vi "Toggle Channel.vi"(8 "error in":errorcluster, 9 "State":bool, 10 "Name":string, 11 "MLTFNC in":refnum<class "MLTFNC.lvclass">) -> (0 "error out":errorcluster, 3 "MLTFNC out":refnum<class "MLTFNC.lvclass">)   [LabVIEW 2019, in "MLTFNC.lvlib" / "MLTFNC.lvclass"]
doc: "This parent method must be called first,\nIt searches for the literal string name of the channel and stores the array index of the literal string if present, or returns an error if the channel is not found."
uses:
  Library/MLTFNC.lvclass
  C:/Users/Public/Documents/Development/builds/Instruments/Instruments.lvlibp/Library/Instruments.lvclass
  builds/Instruments/Instruments.lvlibp/Private/Polymorphic/Special/Event from String.vi
  builds/Instruments/Instruments.lvlibp/Accessors/Command with Logging.vi
  builds/Instruments/Instruments.lvlibp/Library/Instruments.lvclass
  builds/Instruments/Instruments.lvlibp
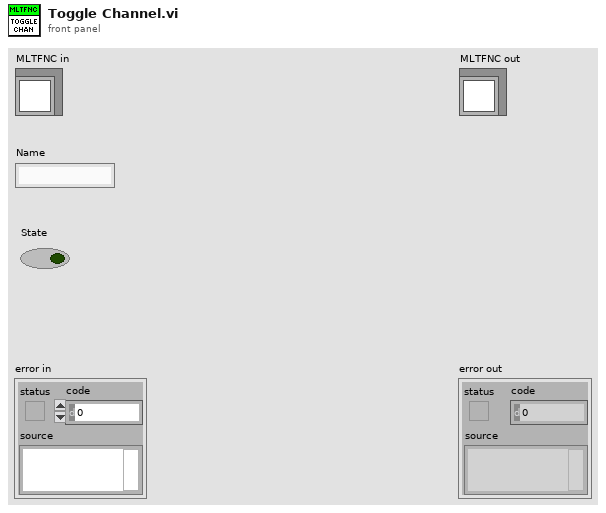
[diagram p1: front panel]
types:
  T1 = cluster{"Timestamp":timestamp, "Description":string, "Data":string}
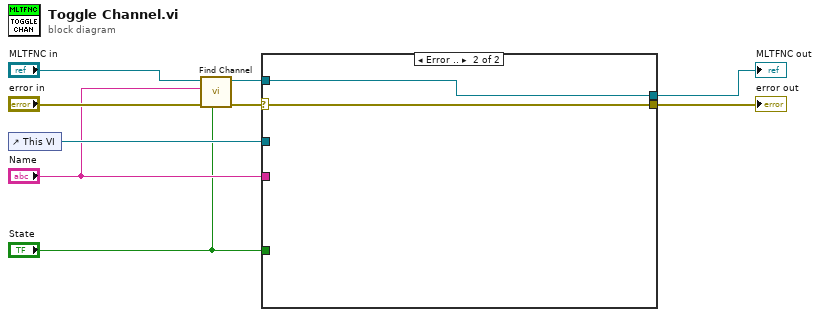
[diagram p0: block diagram]
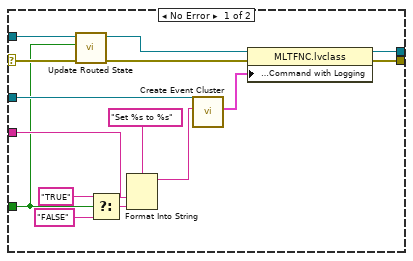
[diagram p2: hidden frame]
diagram:
  n1 = control-ref of="This VI"() -> (w6:refnum<vi>)
  n2 = call "Find Channel.vi"("Set"="State", "error in"="error in", "Name in"="Name", "MLTFNC in"="MLTFNC in") -> ("error out"=w3:errorcluster, "MLTFNC out"=w4:refnum<class "MLTFNC.lvclass">)  [unwired: 6 in]
  n3 = case shown="Error .." w3 {
    selector: w3 -> [w13 w26]
    tunnel: [w24 w26] -> w8
    tunnel: [w23 w25] -> w7
    tunnel: w6 -> [w22 _]
    tunnel: w4 -> [w14 w25]
    tunnel: "Name" -> [w20 _]
    tunnel: "State" -> [w10 _]
    frame No Error {
      n4 = call "Update Routed State.vi"("error in (no error)"=w13, "Set"=w10, "MLTFNC in"=w14) -> ("error out"=w12:errorcluster, "MLTFNC out"=w11:refnum<class "MLTFNC.lvclass">)  [unwired: 7 in]
      n5 = Select(t="TRUE", s=w10, f="FALSE") -> (s? t:f=w17:string)
      n6 = Format Into String(format string="Set %s to %s", w20, w17) -> (resulting string=w18:string)  [unwired: 2 in, 1 out]
      n7 = call-poly "Create Event Cluster.vi"("Value"=w18, "VI Refnum"=w22) -> ("Event Data"=w21:T1)  [unwired: 9 in]
      n8 = property class="MLTFNC.lvclass"(reference=w11, error in=w12, "Accessors:Logging:Command with Logging"=w21) -> (reference out=w23:refnum<class "MLTFNC.lvclass">, error out=w24:errorcluster)
    }
    frame Error {
    }
  }
  "error out" <- w8
  "MLTFNC out" <- w7
